vi "FrequencyAnalysis.vi"(11 "Input":waveform(dbl)[](array[waveform])) -> (3 "Frequencies":dbl[](array[numeric]) format="%.2p")   [LabVIEW 2024]
uses:
  <vilib>/measure/matone.llb/Extract Single Tone Information N Chan.vi
  <vilib>/measure/NI_MAPro.lvlib
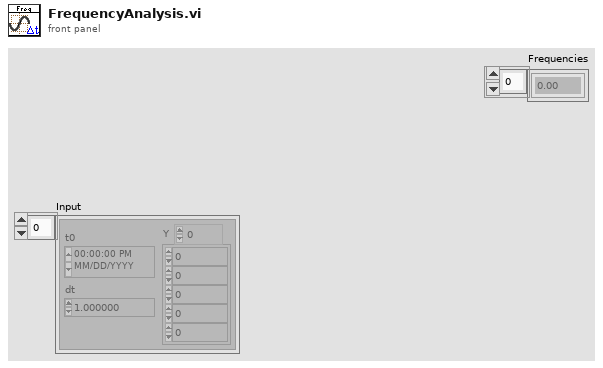
[diagram p1: front panel]
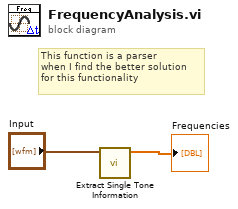
[diagram p0: block diagram]
diagram:
  # "This function is a parser \nwhen I find the better solution \nfor this functionality"
  n1 = call-poly <vilib>:"Extract Single Tone Information.vi"("time signals in"="Input") -> ("detected frequencies"=→"Frequencies":dbl[])  [unwired: 5 in, 5 out]
